vi "ExTestStaticticsI32.vi"() -> ()   [LabVIEW 2010]
panel:
  out "Statistics Bundle":T1 {"Total Area" format="%.2f"; "Centroid Y" format="%.2f"; "Centroid X" format="%.2f"; "Variance" format="%.2f"; "StdDev" format="%.2f"; "Mean Value" format="%.2f"; "Median Value" format="%.2f"; "Max Value" format="%.2f"; "Min Value" format="%.2f"}
  in  "Y Size":i32=100 min=1 max=65535 step=1
  in  "X Size":i32=100 min=1 max=65535 step=1
  out "error out":errorcluster
  in  "error in (no error)":errorcluster
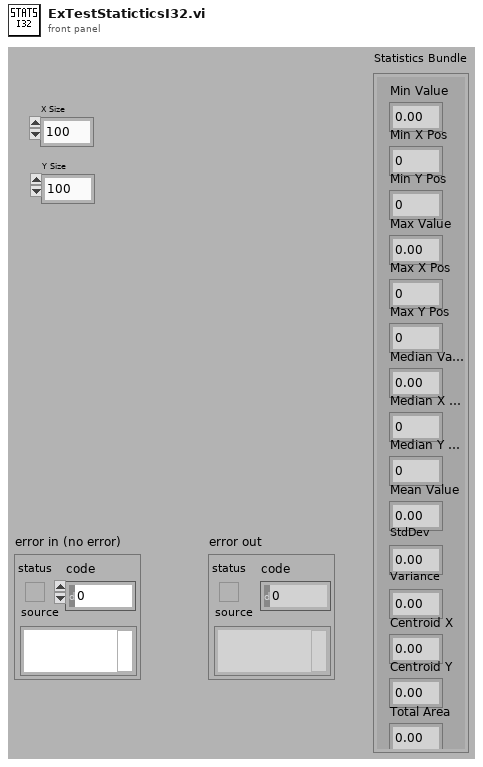
[diagram p1: front panel]
types:
  T1 = cluster{"Min Value":dbl, "Min X Pos":u32, "Min Y Pos":u32, "Max Value":dbl, "Max X Pos":u32, "Max Y Pos":u32, "Median Value":dbl, "Median X Pos":u32, "Median Y Pos":u32, "Mean Value":dbl, "StdDev":dbl, "Variance":dbl, "Centroid X":dbl, "Centroid Y":dbl, "Total Area":dbl}
  T2 = cluster{"Min Value":dbl, "Min X Pos":u32, "Min Y Pos":u32, "Max Value":dbl, "Max X Pos":u32, "Max Y Pos":u32, "Reserved 1":dbl, "Reserved2":u32, "Reserved3":u32, "Mean Value":dbl, "StdDev":dbl, "Variance":dbl, "Centroid X":dbl, "Centroid Y":dbl, "Total Area":dbl}
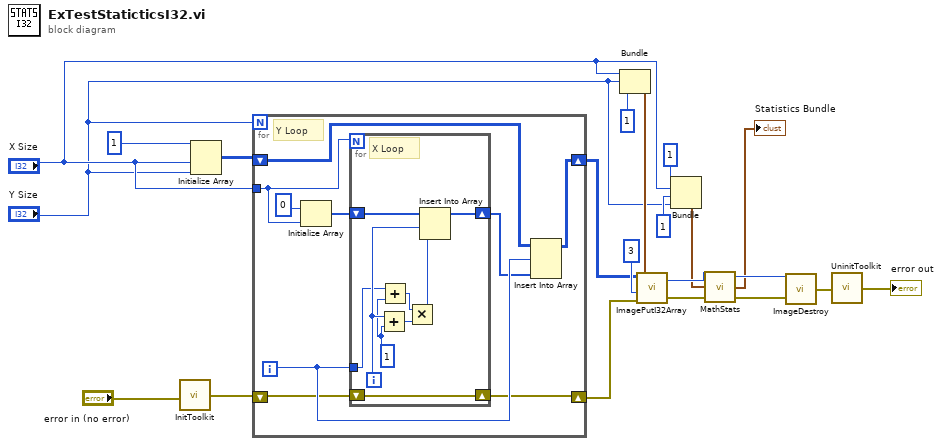
[diagram p0: block diagram]
diagram:
  n1 = call <userlib>:"InitToolkit.vi"("error in"="error in (no error)") -> ("error out"=w3:errorcluster)
  n2 = Initialize Array(1, "X Size", "Y Size") -> (w5:i32[][])
  n3 = for {
    N: "Y Size" -> [_]
    tunnel: "X Size" -> [w30]
    shift-right: [w24] -> w4
    shift-left: w5 -> [w25]
    shift-right: [w22] -> w2
    shift-left: w3 -> [w23]
    i -> [w28]
    # "Y Loop"
    n4 = Initialize Array(0, w30) -> (w27:i32[])
    n5 = for {
      N: w30 -> [_]
      tunnel: w28 -> [w32]
      shift-right: [w35] -> w26
      shift-left: w27 -> [w36]
      shift-right: [w34] -> w22
      shift-left: w23 -> [w34]
      i -> [w39]
      w31 = 1
      # "X Loop"
      n6 = Add(x=w39, y=w31) -> (x+y=w38:i32)
      n7 = Add(x=w32, y=w31) -> (x+y=w33:i32)
      n8 = Multiply(x=w33, y=w38) -> (x*y=w37:i32)
      n9 = Insert Into Array(array=w36, index=w39, new element=w37) -> (w35:i32[])
    }
    n10 = Insert Into Array(array=w25, index (row)=w28, new element=w26) -> (w24:i32[][])  [unwired: 1 in]
  }
  n11 = Bundle("X Size"="X Size", "Y Size"="Y Size", 1) -> (w17:cluster{"X Size":i32, "Y Size":i32, i32})  [unwired: 1 in]
  n12 = call <userlib>:"ImagePutI32Array.vi"("error in (no error)"=w2, "Data Type to store as"=3, "Image dimensions"=w17, "Image Data"=w4) -> ("error out"=w14:errorcluster, "Image Handle"=w12:u32)
  n13 = Bundle(1, "X Size"="X Size", 1, "Y Size"="Y Size") -> (w7:cluster{i32, "X Size":i32, i32, "Y Size":i32})  [unwired: 1 in]
  n14 = call <userlib>:"MathStats.vi"("error in (no error)"=w14, "Region Of Interest bundle"=w7, "Data Handle"=w12) -> ("error out"=w13:errorcluster, "Statistics Bundle"=→"Statistics Bundle":T2, "Data Handle"=w11:u32)
  n15 = call <userlib>:"ImageDestroy.vi"("error in"=w13, "Data handle"=w11) -> ("error out"=w19:errorcluster)
  n16 = call <userlib>:"UninitToolkit.vi"("error in"=w19) -> ("error out"=→"error out":errorcluster)
